vi "Set Channel.vi"(5 "Channel":i32=1 min=1 max=2 step=1, 6 "Channel Status":bool, 7 "Slave":i32=1 min=1 max=6 step=1, 8 "error in (no error)":errorcluster, 11 "VISA resource name":refnum<visa-resource-name>) -> (0 "error out":errorcluster, 3 "VISA resource name out":refnum<visa-resource-name>)   [LabVIEW 2020, in "QuPMXdriver.lvlib"]
doc: "Enable/disable channel."
uses:
  QuPMXdriver.lvlib
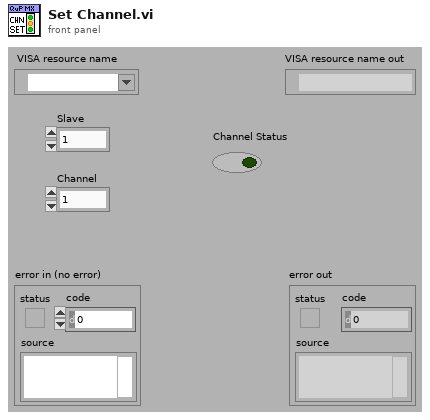
[diagram p1: front panel]
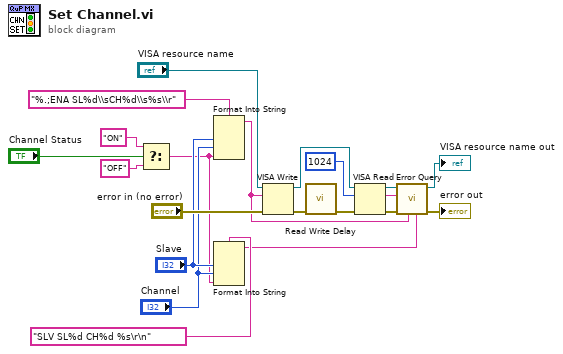
[diagram p0: block diagram]
diagram:
  n1 = Select(t="ON" ("format string"), s="Channel Status", f="OFF" ("format string")) -> (s? t:f=w1:string)
  n2 = Format Into String(format string="%.;ENA SL%d\\sCH%d\\s%s\\r", "Slave", "Channel", w1) -> (resulting string=w9:string)  [unwired: 2 in, 1 out]
  n3 = Format Into String(format string="SLV SL%d CH%d %s\r\n" ("read buffer"), "Slave", "Channel", w1) -> (resulting string=w3:string)  [unwired: 2 in, 1 out]
  n4 = VISA Write(VISA resource name="VISA resource name", write buffer=w9, error in (no error)="error in (no error)") -> (VISA resource name out=w12:refnum<visa-resource-name>, error out=w16:errorcluster)  [unwired: 1 out]
  n5 = call "Read Write Delay.vi"("error in"=w16) -> ("error out"=w15:errorcluster)  [unwired: 10 in]
  n6 = VISA Read(VISA resource name=w12, byte count=u32 1024, error in (no error)=w15) -> (VISA resource name out=w13:refnum<visa-resource-name>, read buffer=w11:string, error out=w10:errorcluster)  [unwired: 1 out]
  n7 = call "Error Query.vi"("Expected read buffer"=w3, "Last command"=w9, "error in (no error)"=w10, "Read buffer"=w11, "VISA resource name"=w13) -> ("error out"=→"error out":errorcluster, "VISA resource name out"=→"VISA resource name out":refnum<visa-resource-name>)  [unwired: 5 in]
